vi "Create Logger.vi"(6 "Debug Level":T1=enum."DEBUG", 8 "error in (no error)":errorcluster, 9 "Sinks":refnum<class "Sink.lvclass">[](array[class]), 10 "Name":string, 11 "Registry in":refnum<class "Registry.lvclass">) -> (0 "error out":errorcluster, 2 "Logger out":refnum<class "Logger.lvclass">, 3 "Registry out":refnum<class "Registry.lvclass">)   [LabVIEW 2020, in "LV Log.lvlib" / "Registry.lvclass"]
uses:
  Registry.lvclass
  Logger/Logger.lvclass
  Sinks/Sink/Sink.lvclass
  Type Defs/Debug Level.ctl
  LV Log.lvlib
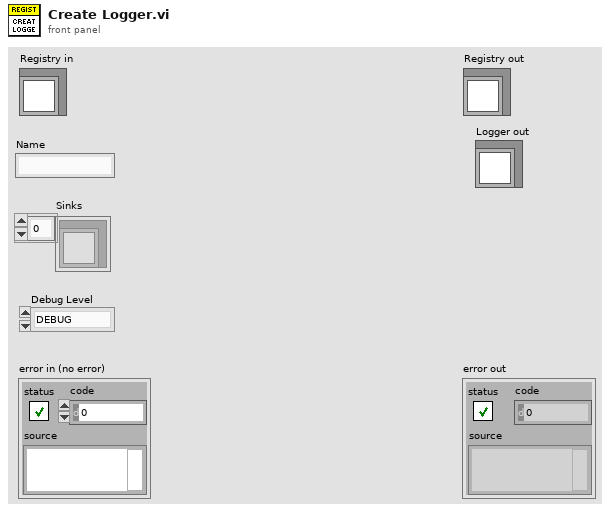
[diagram p1: front panel]
types:
  T1 = typedef "LV Log.lvlib/Debug Level.ctl" = enum16{"DEFAULT", "DEBUG", "INFO", "WARN", "ERROR", "FATAL"}
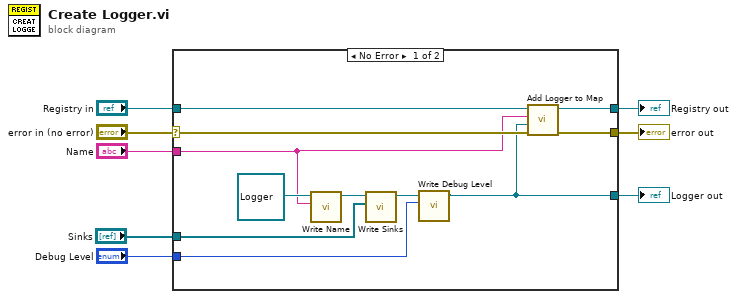
[diagram p0: block diagram]
diagram:
  n1 = case shown="No Error" "error in (no error)" {
    selector: "error in (no error)" -> [w16 w21]
    tunnel: [w15 w21] -> w7
    tunnel: [w17 w20] -> w5
    tunnel: "Registry in" -> [w18 w20]
    tunnel: "Name" -> [w14 _]
    tunnel: [w11 _] -> w3
    tunnel: "Sinks" -> [w10 _]
    tunnel: "Debug Level" -> [w9 _]
    frame No Error {
      n2 = call "Write Name.vi"("Name"=w14, "Logger in"=refnum<class "Logger.lvclass"> refnum ("LV Logging.lvlib:Logger.lvclass")) -> ("Logger out"=w13:refnum<class "Logger.lvclass">)  [unwired: 8 in, 1 out]
      n3 = call "Write Sinks.vi"("Sinks"=w10, "Logger in"=w13) -> ("Logger out"=w12:refnum<class "Logger.lvclass">)  [unwired: 8 in, 1 out]
      n4 = call "Write Debug Level.vi"("Debug Level"=w9, "Logger in"=w12) -> ("Logger out"=w11:refnum<class "Logger.lvclass">)  [unwired: 8 in, 1 out]
      n5 = call "Add Logger to Map.vi"("error in (no error)"=w16, "Logger"=w11, "Name"=w14, "Registry in"=w18) -> ("error out"=w15:errorcluster, "Registry out"=w17:refnum<class "Registry.lvclass">)  [unwired: 6 in]
    }
    frame Error {
    }
  }
  "error out" <- w7
  "Registry out" <- w5
  "Logger out" <- w3
